vi "Disconnect.vi"(8 "error in (no error)":errorcluster, 11 "Simulated Serial Device in":refnum<class "Simulated Serial Device.lvclass">) -> (0 "error out":errorcluster, 3 "Simulated Serial Device out":refnum<class "Simulated Serial Device.lvclass">)   [LabVIEW 2017, in "Simulated Serial Device.lvclass"]
doc: "Disconnect serial port. It is important to execute this code on exit, so the serial port remains available in subsequent runs."
uses:
  Simulated Serial Device.lvclass
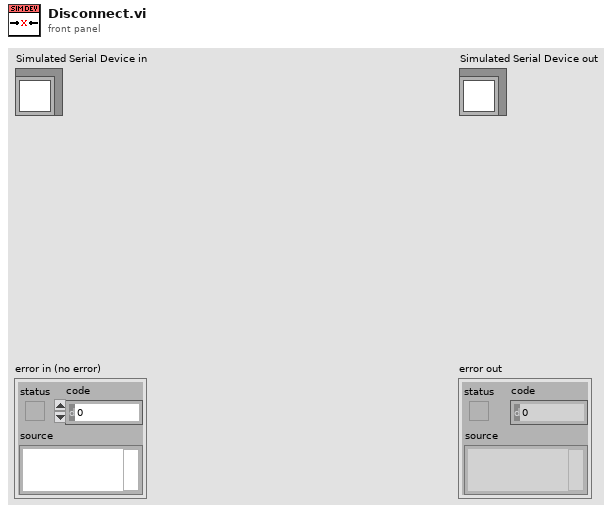
[diagram p1: front panel]
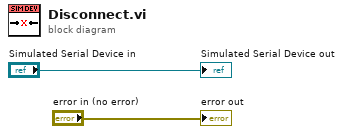
[diagram p0: block diagram]
diagram:
  "error out" <- "error in (no error)"
  "Simulated Serial Device out" <- "Simulated Serial Device in"
